vi "random distribution.vi"(7 "original image":picture[][](array[picture]), 10 "maximumarray width/height":i32, 11 "total array elements":i32) -> (3 "randomisedarray":picture[][](array[picture]))   [LabVIEW 2014]
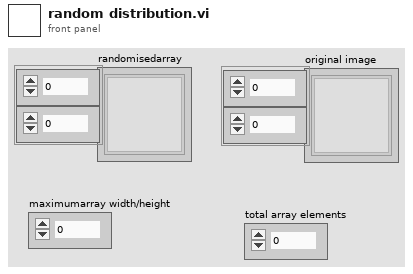
[diagram p1: front panel]
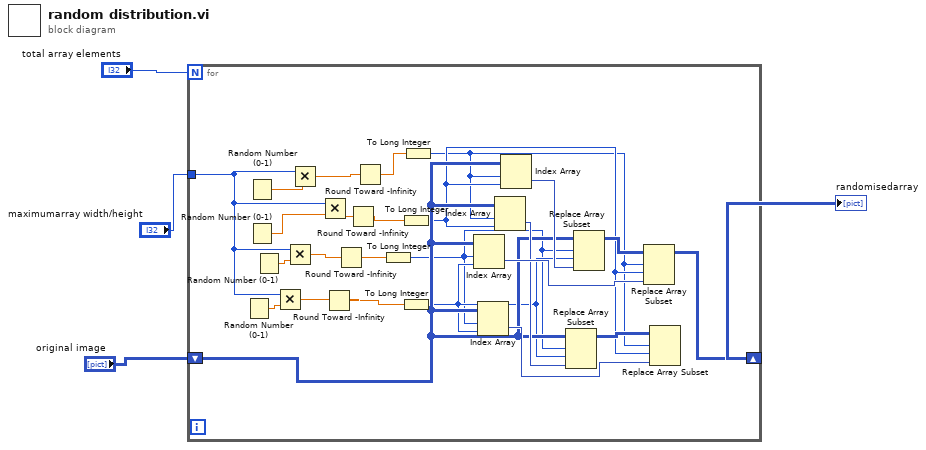
[diagram p0: block diagram]
diagram:
  n1 = for "Shuffle Array Elements" {
    N: "total array elements" -> [_]
    tunnel: "maximumarray width/height" -> [w15]
    shift-right: [w14] -> w2
    shift-left: "original image" -> [w13]
    n2 = Random Number (0-1)() -> (number: 0 to 1=w25:dbl)
    n3 = Random Number (0-1)() -> (number: 0 to 1=w29:dbl)
    n4 = Random Number (0-1)() -> (number: 0 to 1=w26:dbl)
    n5 = Random Number (0-1)() -> (number: 0 to 1=w22:dbl)
    n6 = Multiply(x=w15, y=w25) -> (x*y=w24:dbl)
    n7 = Multiply(x=w15, y=w22) -> (x*y=w23:dbl)
    n8 = Multiply(x=w15, y=w29) -> (x*y=w28:dbl)
    n9 = Multiply(x=w15, y=w26) -> (x*y=w27:dbl)
    n10 = Round Toward -Infinity(1:w24) -> (0:w12:dbl)
    n11 = Round Toward -Infinity(1:w23) -> (0:w10:dbl)
    n12 = Round Toward -Infinity(1:w27) -> (0:w8:dbl)
    n13 = Round Toward -Infinity(1:w28) -> (0:w6:dbl)
    n14 = To Long Integer(number=w10) -> (32bit integer=w9:i32)
    n15 = To Long Integer(number=w8) -> (32bit integer=w7:i32)
    n16 = To Long Integer(number=w12) -> (32bit integer=w11:i32)
    n17 = To Long Integer(number=w6) -> (32bit integer=w5:i32)
    n18 = Index Array(array=w13, index (row)=w9, index (col)=w11) -> (element=w19:picture)
    n19 = Index Array(array=w13, index (row)=w9, index (col)=w11) -> (element=w17:picture)
    n20 = Index Array(array=w13, index (row)=w5, index (col)=w7) -> (element=w16:picture)
    n21 = Index Array(array=w13, index (row)=w5, index (col)=w7) -> (element=w21:picture)
    n22 = Replace Array Subset(array=w13, new element=w16, index (row)=w9, index (col)=w11) -> (w18:picture[][])
    n23 = Replace Array Subset(array=w13, new element=w21, index (row)=w9, index (col)=w11) -> (w20:picture[][])
    n24 = Replace Array Subset(array=w20, new element=w19, index (row)=w5, index (col)=w7) -> (w14:picture[][])
    n25 = Replace Array Subset(array=w18, new element=w17, index (row)=w5, index (col)=w7) -> ()  [unwired: 1 out]
  }
  "randomisedarray" <- w2
